vi "Write OnOff.STS.vi"(8 "error in":errorcluster, 10 "OnOff.STS":bool, 11 "Cycler in":refnum<class "Cycler.lvclass">) -> (0 "error out":errorcluster, 3 "Cycler out":refnum<class "Cycler.lvclass">)   [LabVIEW 2023, in "Cycler.lvclass"]
uses:
  Cycler.lvclass
  Cycler.lvclass/Cycler.ctl
  <vilib>/ADAS Replay HIL/Channels/Tag Wrapper/Tag Wrapper.lvlib
  <vilib>/ADAS Replay HIL/Channels/Tag Wrapper/Polymorphic/Write Channel (Boolean).vi
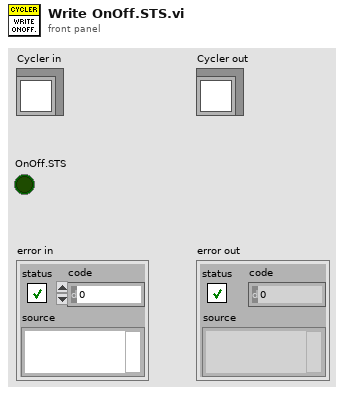
[diagram p1: front panel]
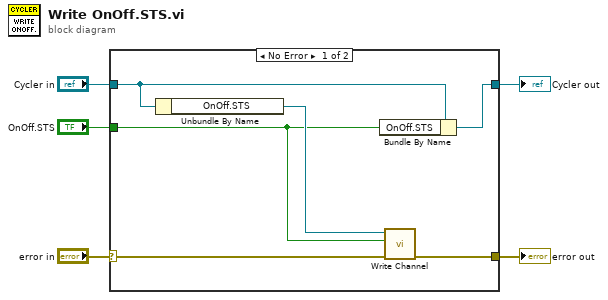
[diagram p0: block diagram]
diagram:
  n1 = case shown="No Error" "error in" {
    selector: "error in" -> [w9 w12]
    tunnel: [w8 w12] -> w4
    tunnel: [w11 w13] -> w2
    tunnel: "Cycler in" -> [w10 w13]
    tunnel: "OnOff.STS" -> [w6 _]
    frame No Error {
      n2 = Unbundle By Name(w10) -> ("OnOff.STS"=w7:refnum<k21>)
      n3 = Bundle By Name(cluster=w10, "OnOff.STS"=w6) -> (w11:refnum<class "Cycler.lvclass">)
      n4 = call-poly <vilib>:"Write Channel.vi"("error in"=w9, "Value to Write"=w6, "ADAS HIL Channel in"=w7) -> ("error out"=w8:errorcluster)  [unwired: 6 in, 2 out]
    }
    frame Error {
    }
  }
  "error out" <- w4
  "Cycler out" <- w2
